vi "Pre Launch Init.vi"(11 "Work Dispatcher in":refnum<class "Work Dispatcher.lvclass">) -> (0 "error out":errorcluster, 3 "Work Dispatcher out":refnum<class "Work Dispatcher.lvclass">)   [LabVIEW 2023, in "Work Dispatcher.lvlib" / "Work Dispatcher.lvclass"]
doc: "(<B>Filename</B>: Actor Framework.lvlib:Actor.lvclass:Pre Launch Init.vi)\n\nDefines behavior that occurs after the Launch Nested Actor method is invoked but before the actor's Actor Core method begins running.\n\nBy default, this method does nothing. A descendant class may override it to define behavior."
uses:
  Work Dispatcher.lvclass
  <vilib>/ActorFramework/Message Enqueuer/Message Enqueuer.lvclass
  Work Dispatcher.lvclass/Work Dispatcher.ctl
  <vilib>/ActorFramework/Actor/Actor.lvclass
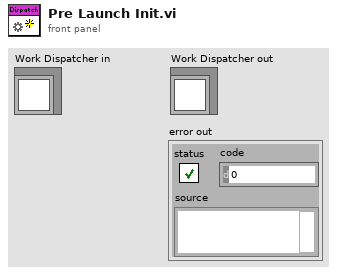
[diagram p1: front panel]
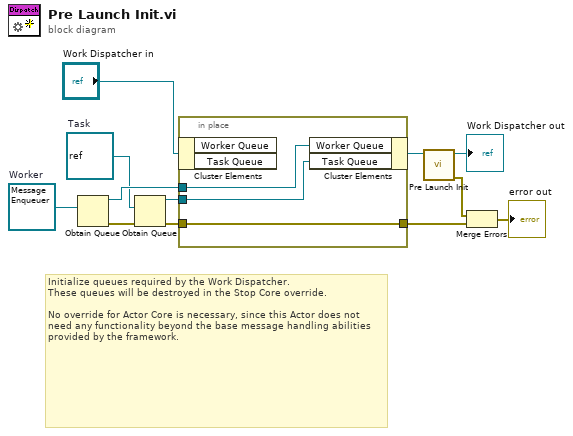
[diagram p0: block diagram]
diagram:
  w9 = refnum<class "Message Enqueuer.lvclass"> refnum  # Worker
  w7 = refnum<class> refnum  # Task
  # "Initialize queues required by the Work Dispatcher.  \nThese queues will be destroyed in the Stop Core override.\n\nNo override for Actor Core is necessary, since this Actor does not need any functionality beyond the base message handling abilities provided by the framework."
  n1 = Obtain Queue(element data type=w9) -> (queue out=w10:refnum<queue>, error out=w6:errorcluster)  [unwired: 4 in, 1 out]
  n2 = Obtain Queue(element data type=w7, error in (no error)=w6) -> (queue out=w8:refnum<queue>, error out=w11:errorcluster)  [unwired: 3 in, 1 out]
  n3 = in-place {
    in-place-border: w8 -> [w15]
    in-place-border: w10 -> [w14]
    in-place-border: w11 -> [w13]
    in-place-border: [w13] -> w3
    n4 = in-place-cluster #1("Work Dispatcher in") -> ()  [unwired: 2 out]
    n5 = in-place-cluster #1("Worker Queue"=w14, "Task Queue"=w15) -> (w12:refnum<class "Work Dispatcher.lvclass">)
  }
  n6 = call-parent "Pre Launch Init.vi"("Actor in"=w12) -> ("error out"=w4:errorcluster, "Actor out"=→"Work Dispatcher out":refnum<class "Work Dispatcher.lvclass">)  [unwired: 9 in]
  n7 = Merge Errors(w4, w3) -> (→"error out":errorcluster)
